vi "cancel.vi"(8 "error in":errorcluster, 11 "cancel token in":refnum<class "cancel token.lvclass">) -> (0 "error out":errorcluster, 3 "cancel token out":refnum<class "cancel token.lvclass">)   [LabVIEW 2013, in "cancel token.lvclass"]
uses:
  cancel token.lvclass
  cancel token.lvclass/cancel token.ctl
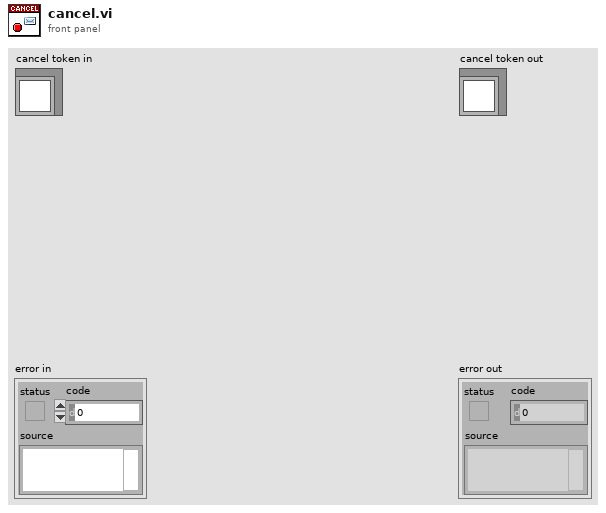
[diagram p1: front panel]
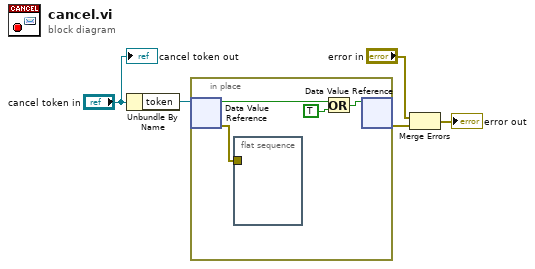
[diagram p0: block diagram]
diagram:
  n1 = Unbundle By Name("cancel token in") -> ("token"=w3:refnum<data-value>)
  n2 = in-place {
    n3 = in-place-dvr #1(w3) -> (w7:bool, w6:errorcluster)
    n4 = flat-sequence {
      tunnel: w6 -> [_]
      frame #0 {
      }
    }
    n5 = Or(x=w7, y=TRUE) -> (x .or. y?=w8:bool)
    n6 = in-place-dvr #1(w8) -> (w1:errorcluster)  [unwired: 1 out]
  }
  n7 = Merge Errors("error in", w1) -> (→"error out":errorcluster)
  "cancel token out" <- "cancel token in"
